vi "Read Compass Data.vi"(8 "error in (no error)":errorcluster, 11 "Simulator in":refnum<class "Simulator.lvclass">) -> (0 "error out":errorcluster, 2 "Compass Reading":dbl, 3 "Simulator out":refnum<class "Simulator.lvclass">)   [LabVIEW 2011, in "Simulator.lvclass"]
uses:
  Simulator.lvclass
  Simulator.lvclass/Simulator.ctl
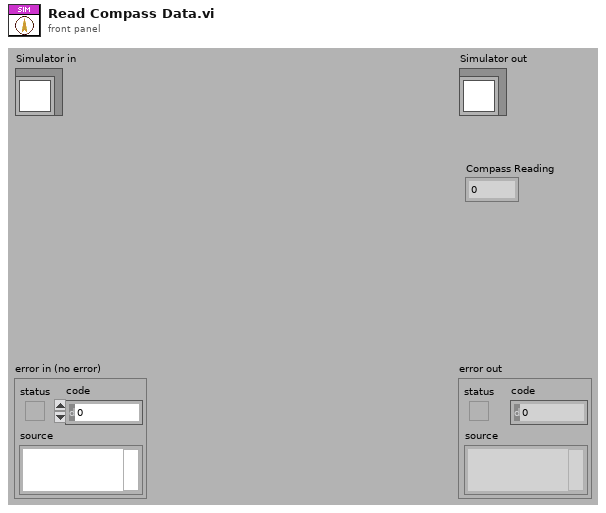
[diagram p1: front panel]
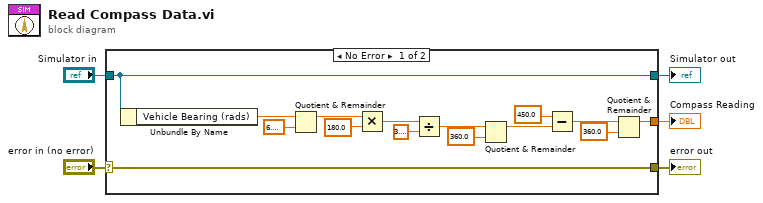
[diagram p0: block diagram]
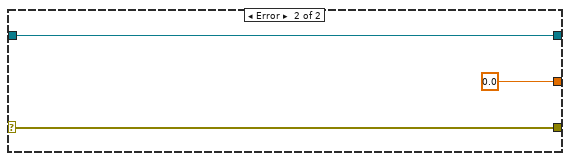
[diagram p2: hidden frame]
diagram:
  n1 = case shown="No Error" "error in (no error)" {
    selector: "error in (no error)" -> [w20 w23]
    tunnel: [w20 w23] -> w4
    tunnel: [w19 w22] -> w2
    tunnel: "Simulator in" -> [w19 w22]
    tunnel: [w12 0.0] -> w1
    frame No Error {
      n2 = Unbundle By Name(w19) -> ("Vehicle Bearing (rads)"=w7:dbl)
      n3 = Quotient & Remainder(x=w7, y=6.283185307179586) -> (x-y*floor(x/y)=w8:dbl)  [unwired: 1 out]
      n4 = Multiply(x=w8, y=180.0) -> (x*y=w17:dbl)
      n5 = Divide(x=w17, y=3.141592653589793) -> (x/y=w6:dbl)
      n6 = Quotient & Remainder(x=w6, y=360.0) -> (x-y*floor(x/y)=w11:dbl)  [unwired: 1 out]
      n7 = Subtract(x=450.0, y=w11) -> (x-y=w14:dbl)
      n8 = Quotient & Remainder(x=w14, y=360.0) -> (x-y*floor(x/y)=w12:dbl)  [unwired: 1 out]
    }
    frame Error {
    }
  }
  "error out" <- w4
  "Simulator out" <- w2
  "Compass Reading" <- w1
